vi "TIFF File Reader (LAVA.org).vi"(0 "Input Image":string) -> (3 "Grayscale":picture, 4 "Gray16/32":sgl[][](array[numeric]), 5 "Gray8":u8[][](array[numeric]), 7 "Gray u16":u16[][](array[numeric]))   [LabVIEW 2014]
doc: "This SubVI is an optimized version of the VI Load Flattened Image from Tiff.vi created by Gavin Burnell and Herbert Looser\n\nFiles in this folder downloaded from http://code.google.com/p/lavacr/source/browse/#svn/trunk/8.5.x/Machine%20Vision%20and%20Imaging/TIFF%20File%20Reader (free download).\nSee the discussion on https://lavag.org/topic/7170-tiff-reader/, where the link to above repository was provided.\nPeter Buerki, January 19, 2015."
uses:
  SubVIs/Globals.vi
  LAVA TIFF File Reader.lvlib
panel:
  out "Post View Image (NO IMAQ)":sgl[][](graph)
  in  "Tab Control":T1(tab)
  out "N_Bits":u64
  out "GrayWithLUT":picture
  out "Gray8 LUT":u8[][](array[numeric])
  out "RGB":picture
  out "N_RGB_Bits":u64
  out "R16/32":sgl[][](array[numeric])
  out "G16/32":sgl[][](array[numeric])
  out "B16/32":sgl[][](array[numeric])
  out "RGB8":u32[][](array[numeric])
  out "PhotoM":T2(ring)=enum."BlackIsZero"
  # "HD1:\\Users\\herbertlooser\\Desktop\\LadungssprŸher.tif"
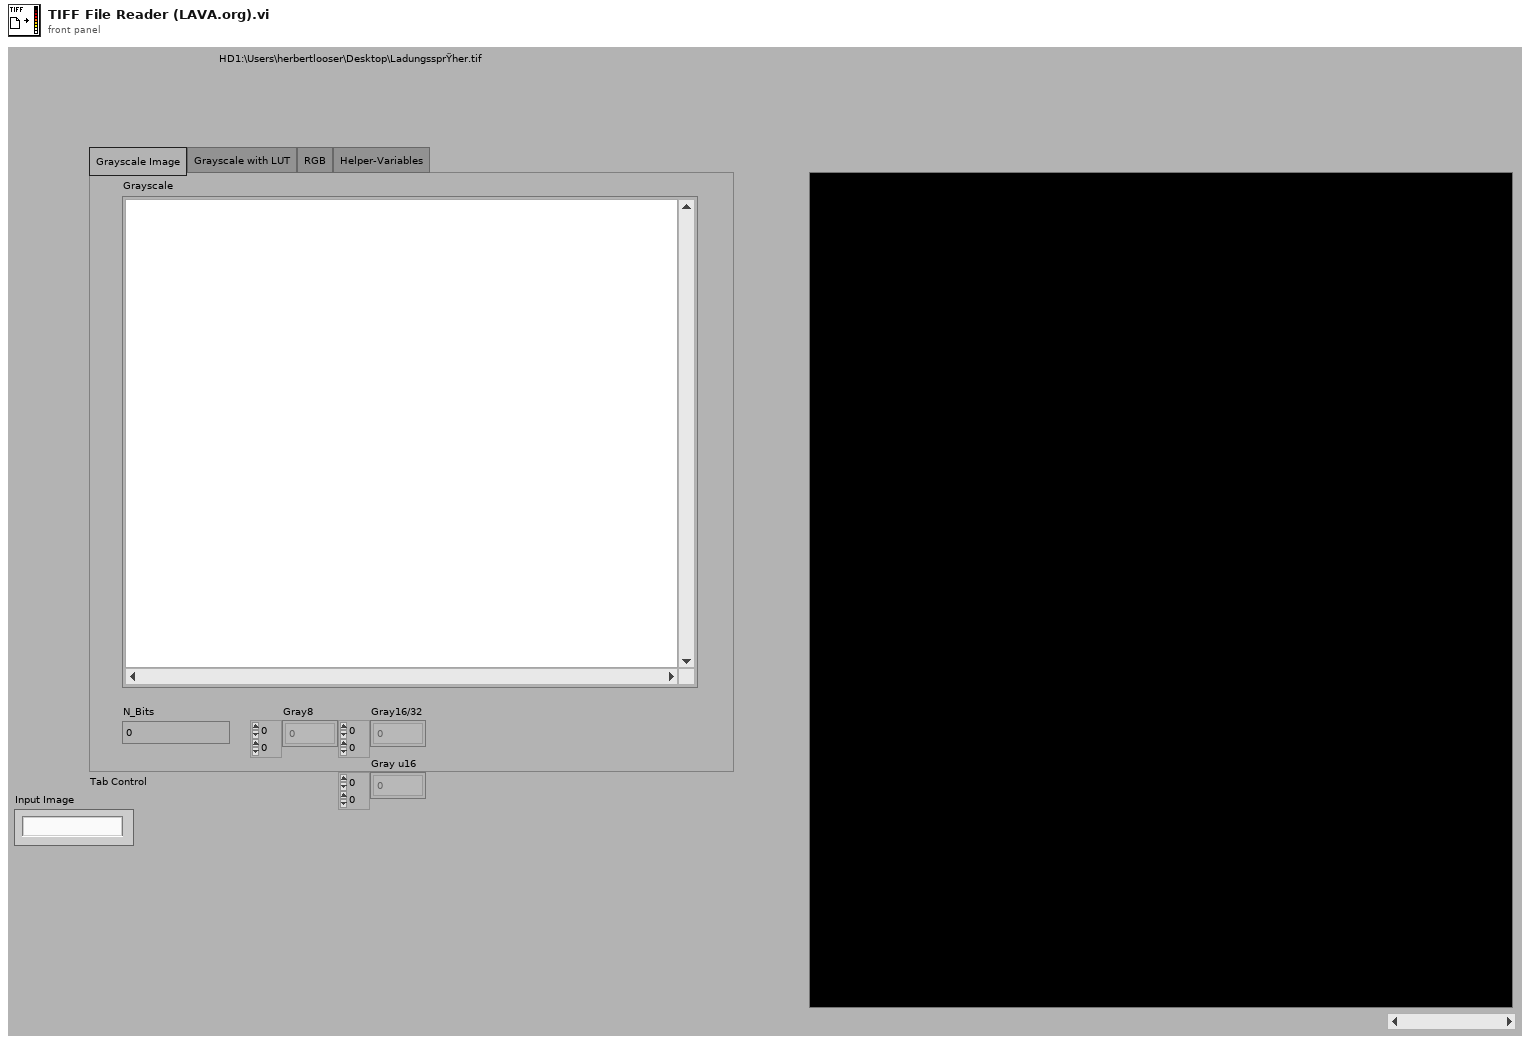
[diagram p1: front panel]
types:
  T1 = enum32{"Grayscale Image", "Grayscale with LUT", "RGB", "Helper-Variables"}
  T2 = enum16{"WhiteIsZero", "BlackIsZero", "RGB", "RGBPalette", "TranspMask", "CMYK", "YCbCr", "Null", "CIELab"}
  T3 = typedef "LAVA TIFF File Reader.lvlib/IFD Entry.ctl" = cluster{"Tag":u16, "Type":T4, "Count":u32, "Val/Offs":u32, "Is Val/Offs(T)":bool}
  T4 = typedef "LAVA TIFF File Reader.lvlib/FieldTypes.ctl" = enum16{"NULL", "U8", "ASCII7", "U16", "U32", "RATIONAL", "SByte(I8)", "Undef(8Bit)", "I16", "I32", "SRat(4B:4B)", "SGL(4Byte)", "DBL(8Byte)"}
  T5 = typedef "imagedata.ctl" = cluster{"image type":i32, "image depth":i32, "image":u8[], "mask":u8[], "colors":u32[], "Rectangle":cluster{"left":i16, "top":i16, "right":i16, "bottom":i16}}
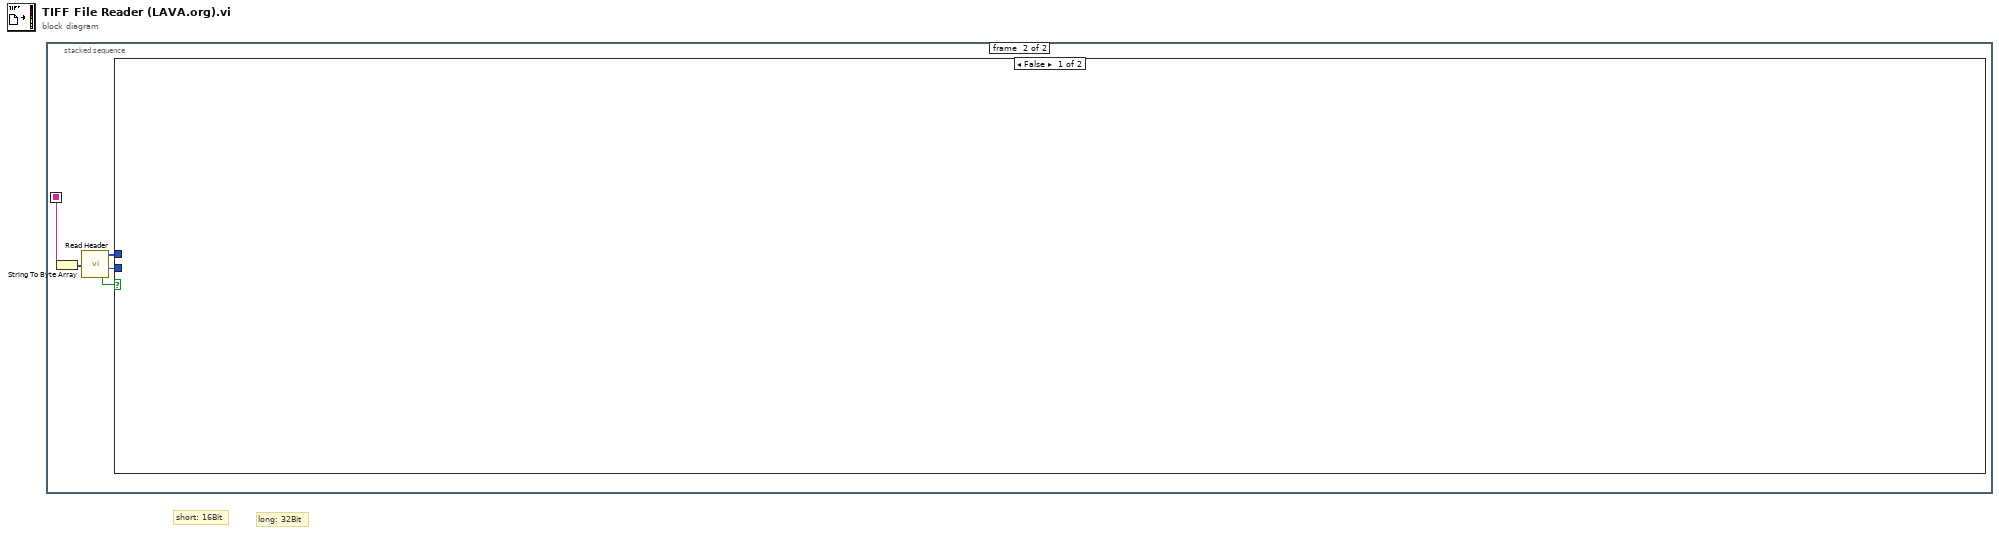
[diagram p0: block diagram]
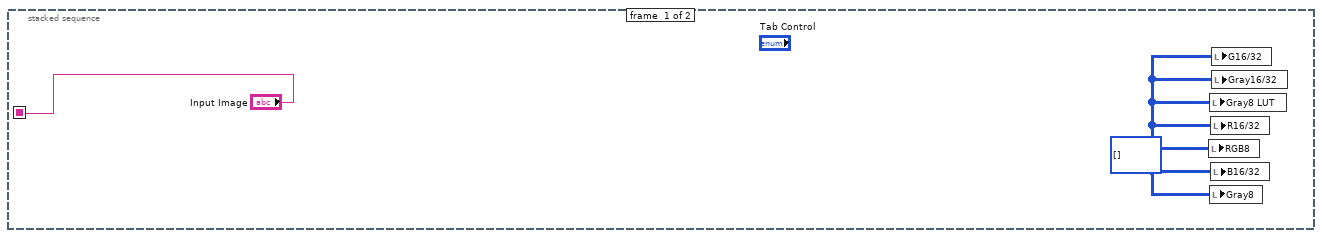
[diagram p2: hidden frame]
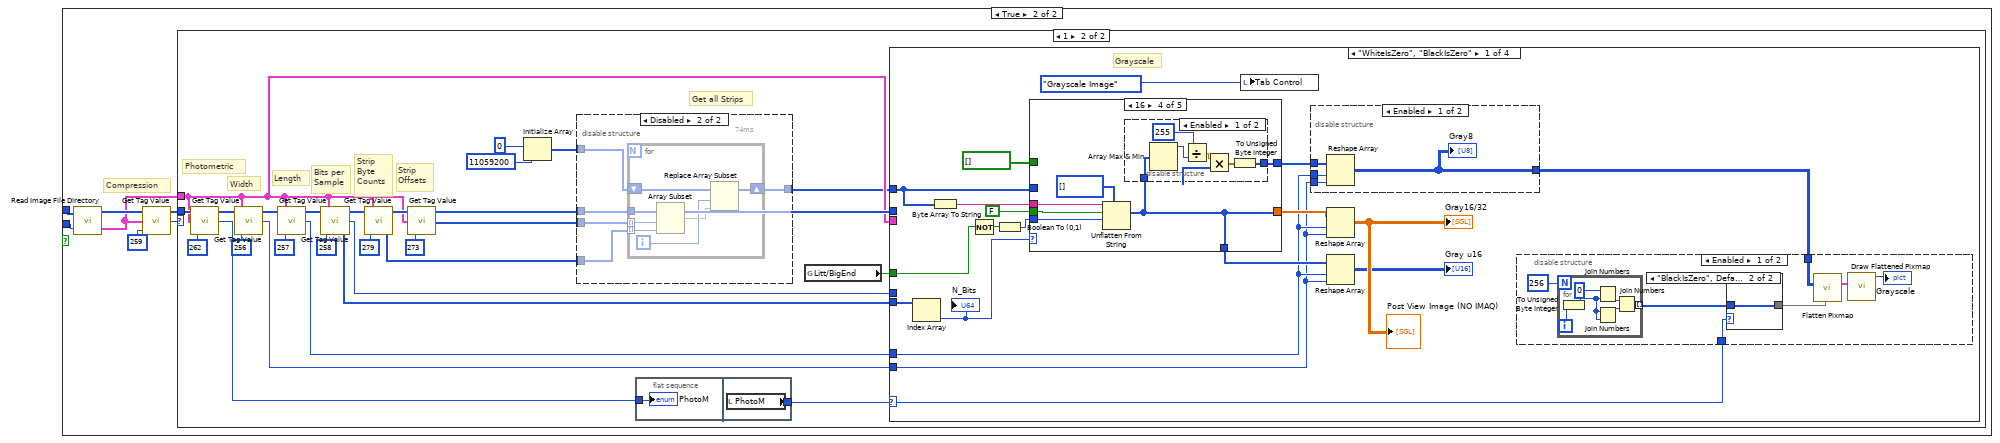
[diagram p3: hidden frame]
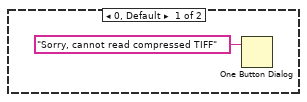
[diagram p4: hidden frame]
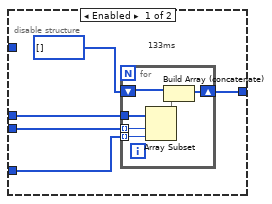
[diagram p5: hidden frame]
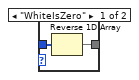
[diagram p7: hidden frame]
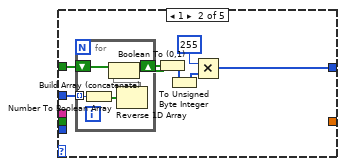
[diagram p10: hidden frame]
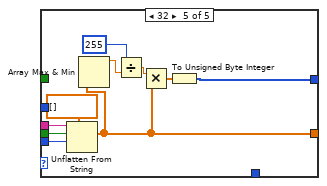
[diagram p13: hidden frame]
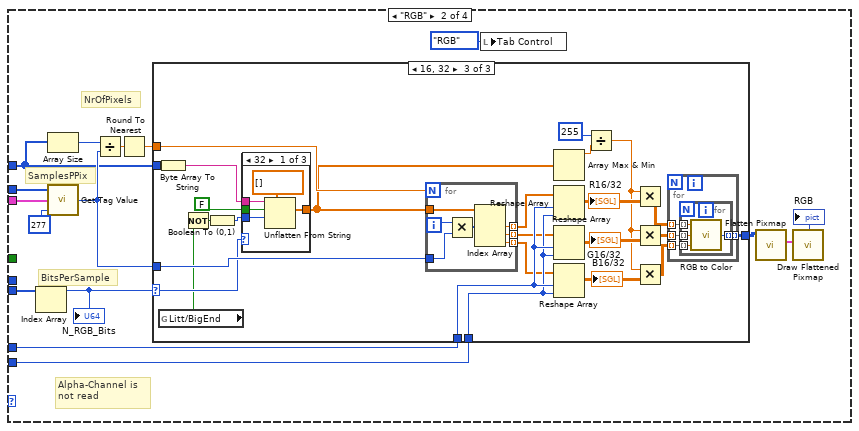
[diagram p14: hidden frame]
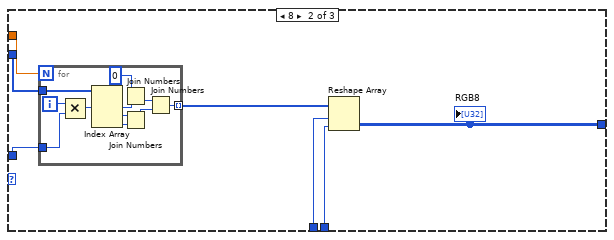
[diagram p16: hidden frame]
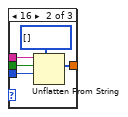
[diagram p17: hidden frame]
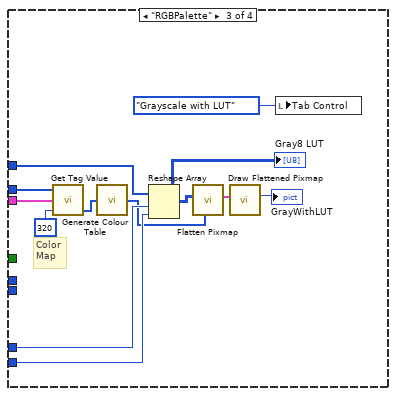
[diagram p19: hidden frame]
diagram:
  # "long: 32Bit"
  # "short: 16Bit"
  n1 = stacked-sequence {
    seq-local: ["Input Image" _] -> [_ w6]
    frame #0 {
      w2 = u32[][] [] ("RGB8")
      n2 = local write "RGB8"(w2) -> ()
      n3 = local write "Gray8 LUT"(w2) -> ()
      n4 = local write "Gray8"(w2) -> ()
      n5 = local write "R16/32"(w2) -> ()
      n6 = local write "B16/32"(w2) -> ()
      n7 = local write "G16/32"(w2) -> ()
      n8 = local write "Gray16/32"(w2) -> ()
    }
    frame #1 {
      n9 = String To Byte Array(string=w6) -> (unsigned byte array=w7:u8[])
      n10 = call "Read Header.vi"("Image Data in"=w7) -> ("Image Data out"=w5:u8[], "ImFileDirectOffs"=w4:u32, "isTIFF"=w3:bool)  [unwired: 1 in]
      n11 = case shown="False" w3 {
        tunnel: w5 -> [_ w13]
        tunnel: w4 -> [_ w12]
        frame False {
        }
        frame True {
          # "Compression"
          n12 = call "Read Image File Directory.vi"("Im_File_Dir Offs"=w12, "Image Data in"=w13) -> ("Directory"=w8:T3[], "Image Data out"=w11:u8[])
          n13 = call "Get Tag Value.vi"("Tag Code"=u16 259, "DirEntries"=w8) -> ("Single Value"=w9:u32)  [unwired: 1 in, 2 out]
          n14 = case shown="1" w9 {
            tunnel: w11 -> [_ w36]
            tunnel: w8 -> [_ w20]
            frame 0, Default {
              n15 = One Button Dialog(message="Sorry, cannot read compressed TIFF") -> ()  [unwired: 1 in, 1 out]
            }
            frame 1 {
              # "Get all Strips"
              # "Strip\nOffsets"
              # "Strip\nByte\nCounts"
              # "Bits per\nSample"
              # "Photometric"
              # "Length"
              # "Width"
              n16 = call "Get Tag Value.vi"("Tag Code"=u16 262, "DirEntries"=w20, "Image Data in"=w36) -> ("Single Value"=w25:u32, "Image Data out"=w35:u8[])  [unwired: 1 out]
              n17 = call "Get Tag Value.vi"("Tag Code"=u16 256, "DirEntries"=w20, "Image Data in"=w35) -> ("Single Value"=w37:u32, "Image Data out"=w41:u8[])  [unwired: 1 out]
              n18 = call "Get Tag Value.vi"("Tag Code"=u16 257, "DirEntries"=w20, "Image Data in"=w41) -> ("Single Value"=w38:u32, "Image Data out"=w32:u8[])  [unwired: 1 out]
              n19 = call "Get Tag Value.vi"("Tag Code"=u16 258, "DirEntries"=w20, "Image Data in"=w32) -> ("Multiple Values"=w26:u64[], "Single Value"=w27:u32, "Image Data out"=w31:u8[])
              n20 = call "Get Tag Value.vi"("Tag Code"=u16 279, "DirEntries"=w20, "Image Data in"=w31) -> ("Multiple Values"=w21:u64[], "Image Data out"=w30:u8[])  [unwired: 1 out]
              n21 = call "Get Tag Value.vi"("Tag Code"=u16 273, "DirEntries"=w20, "Image Data in"=w30) -> ("Multiple Values"=w22:u64[], "Image Data out"=w23:u8[])  [unwired: 1 out]
              n22 = Initialize Array(u8 0 ("Numeric"), 11059200 ("dimension size")) -> (w16:u8[])
              n23 = disable-structure shown="Disabled" {
                disable-tunnel: w23 -> [w46 w57]
                disable-tunnel: w22 -> [w45 w56]
                disable-tunnel: w21 -> [w44 w55]
                disable-tunnel: [w42 w54] -> w18
                disable-tunnel: w16 -> [_ w53]
                frame Enabled {
                  # "133ms"
                  n24 = for {
                    tunnel: w46 -> [w52]
                    tunnel: w45 -> [w51] mode=indexing
                    tunnel: w44 -> [w50] mode=indexing
                    shift-right: [w49] -> w42
                    shift-left: u8[] [] -> [w47]
                    n25 = Array Subset(array=w52, index=w51, length=w50) -> (w48:u8[])
                    n26 = Build Array (concatenate)(w47, w48) -> (w49:u8[])
                  }
                }
                frame Disabled {
                  # "74ms"
                  n27 = for {
                    tunnel: w57 -> [w64]
                    tunnel: w56 -> [w63] mode=indexing
                    tunnel: w55 -> [w62] mode=indexing
                    shift-right: [w60] -> w54
                    shift-left: w53 -> [w61]
                    i -> [w59]
                    n28 = Array Subset(array=w64, index=w63, length=w62) -> (w58:u8[])
                    n29 = Replace Array Subset(array=w61, new element=w58, index=w59) -> (w60:u8[])
                  }
                }
              }
              n30 = flat-sequence {
                tunnel: w25 -> [w65]
                tunnel: [w66] -> w24
                frame #0 {
                  "PhotoM" <- w65
                }
                frame #1 {
                  n31 = local read "PhotoM"() -> (w66:T2)
                }
              }
              n32 = global read "Globals.vi" "Litt/BigEnd"() -> (w19:bool)
              n33 = case shown="\"WhiteIsZero\", \"BlackIsZero\"" w24 {
                selector: w24 -> [w77 _ _ _]
                tunnel: w38 -> [w68 w156 w231 _]
                tunnel: w23 -> [_ w154 w233 _]
                tunnel: w37 -> [w67 w155 w230 _]
                tunnel: w20 -> [_ w153 w236 _]
                tunnel: w27 -> [_ _ _ _]
                tunnel: w26 -> [w81 w151 _ _]
                tunnel: w18 -> [w80 w142 w229 _]
                tunnel: w19 -> [w74 _ _ _]
                frame "WhiteIsZero", "BlackIsZero" {
                  # "Grayscale"
                  n34 = Index Array(array=w81) -> (element=w76:u64)  [unwired: 1 in]
                  "N_Bits" <- w76
                  n35 = Byte Array To String(unsigned byte array=w80) -> (string=w85:string)
                  n36 = Not(x=w74) -> (.not. x?=w82:bool)
                  n37 = Boolean To (0,1)(Boolean=w82) -> (0, 1=w83:i16)
                  n38 = case shown="16" w76 {
                    tunnel: w85 -> [_ _ _ w124 w139]
                    tunnel: [_ _ w118 w119 w132] -> w78
                    tunnel: FALSE ("data includes array or string size? (T)") -> [_ _ _ w123 w138]
                    tunnel: w83 -> [_ _ _ w122 w137]
                    tunnel: w80 -> [_ w112 w118 _ _]
                    tunnel: [_ w107 w118 w120 w133] -> w79
                    tunnel: bool[] [] -> [_ w106 _ _ _]
                    tunnel: [_ _ _ w119 _] -> w69
                    frame 0, 4, Default {
                      # "not\nsupported"
                    }
                    frame 1 {
                      n39 = for {
                        tunnel: w112 -> [w117] mode=indexing
                        shift-right: [w116] -> w111
                        shift-left: w106 -> [w115]
                        n40 = Number To Boolean Array(number=w117) -> (Boolean array=w114:bool[])
                        n41 = Reverse 1D Array(array=w114) -> (reversed array=w113:bool[])
                        n42 = Build Array (concatenate)(w115, w113) -> (w116:bool[])
                      }
                      n43 = Boolean To (0,1)(Boolean=w111) -> (0, 1=w110:i16[])
                      n44 = To Unsigned Byte Integer(number=w110) -> (unsigned 8bit integer=w109:u8[])
                      n45 = Multiply(x=u8 255, y=w109) -> (x*y=w107:u8[])
                    }
                    frame 8 {
                    }
                    frame 16 {
                      n46 = Unflatten From String(type=u16[] [], binary string=w124, data includes array or string size? (T)=w123, byte order (0:big-endian, network order)=w122) -> (value=w119:u16[])  [unwired: 1 in, 2 out]
                      n47 = disable-structure shown="Enabled" {
                        disable-tunnel: [w126 _] -> w120
                        disable-tunnel: w119 -> [w125 _]
                        frame Enabled {
                          n48 = Array Max & Min(array=w125) -> (max value=w130:u16)  [unwired: 3 out]
                          n49 = Divide(x=255 ("Numeric"), y=w130) -> (x/y=w129:dbl)
                          n50 = Multiply(x=w129, y=w125) -> (x*y=w127:dbl[])
                          n51 = To Unsigned Byte Integer(number=w127) -> (unsigned 8bit integer=w126:u8[])
                        }
                        frame Disabled {
                        }
                      }
                    }
                    frame 32 {
                      n52 = Unflatten From String(type=sgl[] [], binary string=w139, data includes array or string size? (T)=w138, byte order (0:big-endian, network order)=w137) -> (value=w132:sgl[])  [unwired: 1 in, 2 out]
                      n53 = Array Max & Min(array=w132) -> (max value=w136:sgl)  [unwired: 3 out]
                      n54 = Divide(x=255 ("Numeric"), y=w136) -> (x/y=w135:sgl)
                      n55 = Multiply(x=w135, y=w132) -> (x*y=w134:sgl[])
                      n56 = To Unsigned Byte Integer(number=w134) -> (unsigned 8bit integer=w133:u8[])
                    }
                  }
                  n57 = local write "Tab Control"(T1."Grayscale Image" ("Tab Control")) -> ()
                  n58 = disable-structure shown="Enabled" {
                    disable-tunnel: w79 -> [w89 _]
                    disable-tunnel: w68 -> [w88 _]
                    disable-tunnel: w67 -> [w87 _]
                    disable-tunnel: [w86 _] -> w72
                    frame Enabled {
                      n59 = Reshape Array(w89, w88, w87) -> (w86:u8[][])
                      "Gray8" <- w86
                    }
                    frame Disabled {
                    }
                  }
                  n60 = Reshape Array(w78, w68, w67) -> (→"Gray16/32" →"Post View Image (NO IMAQ)":sgl[][])
                  n61 = Reshape Array(w69, w68, w67) -> (→"Gray u16":u16[][])
                  n62 = disable-structure shown="Enabled" {
                    disable-tunnel: w77 -> [w92 _]
                    disable-tunnel: w72 -> [w90 _]
                    frame Enabled {
                      n63 = for {
                        N: 256 -> [_]
                        tunnel: [w100] -> w94 mode=indexing
                        i -> [w105]
                        n64 = To Unsigned Byte Integer(number=w105) -> (unsigned 8bit integer=w103:u8)
                        n65 = Join Numbers(hi=u8 0, lo=w103) -> ((hi.lo)=w101:u16)
                        n66 = Join Numbers(hi=w103, lo=w103) -> ((hi.lo)=w102:u16)
                        n67 = Join Numbers(hi=w101, lo=w102) -> ((hi.lo)=w100:u32)
                      }
                      n68 = case shown="\"BlackIsZero\", Default" w92 {
                        tunnel: w94 -> [w98 w99]
                        tunnel: [w97 w99] -> w93
                        frame "WhiteIsZero" {
                          n69 = Reverse 1D Array(array=w98) -> (reversed array=w97:u32[])
                        }
                        frame "BlackIsZero", Default {
                        }
                      }
                      n70 = call <vilib>:"Flatten Pixmap.vi"("colors"=w93, "8-bit pixmap"=w90) -> ("image data"=w96:T5)  [unwired: 9 in]
                      n71 = call <vilib>:"Draw Flattened Pixmap.vi"("image data"=w96) -> ("new picture"=→"Grayscale":picture)  [unwired: 8 in]
                    }
                    frame Disabled {
                    }
                  }
                }
                frame "RGB" {
                  # "BitsPerSample"
                  # "NrOfPixels"
                  # "Alpha-Channel is\nnot read"
                  # "SamplesPPix"
                  n72 = Index Array(array=w151) -> (element=w146:u64)  [unwired: 1 in]
                  "N_RGB_Bits" <- w146
                  n73 = Array Size(array=w142) -> (size(s)=w141:i32)
                  n74 = call "Get Tag Value.vi"("Tag Code"=u16 277, "DirEntries"=w153, "Image Data in"=w154) -> ("Single Value"=w148:u32)  [unwired: 2 out]
                  n75 = Divide(x=w141, y=w148) -> (x/y=w150:dbl)
                  n76 = Round To Nearest(number=w150) -> (nearest integer value=w149:dbl)
                  n77 = case shown="16, 32" w146 {
                    selector: w146 -> [_ _ w191]
                    tunnel: w156 -> [_ w162 w199]
                    tunnel: w155 -> [_ w161 w198]
                    tunnel: w148 -> [_ w160 w195]
                    tunnel: w142 -> [_ w159 w190]
                    tunnel: w149 -> [_ w158 w196]
                    tunnel: [_ w157 w176] -> w143
                    frame 0, Default {
                    }
                    frame 8 {
                      n78 = for {
                        N: w158 -> [_]
                        tunnel: w159 -> [w174]
                        tunnel: [w167] -> w163 mode=indexing
                        tunnel: w160 -> [w164]
                        i -> [w165]
                        n79 = Multiply(x=w165, y=w164) -> (x*y=w166:u32)
                        n80 = Index Array(array=w174, index #1=w166) -> (element #1=w173:u8, element #2=w172:u8, element #3=w171:u8)  [unwired: 2 in]
                        n81 = Join Numbers(hi=u8 0, lo=w173) -> ((hi.lo)=w168:u16)
                        n82 = Join Numbers(hi=w172, lo=w171) -> ((hi.lo)=w169:u16)
                        n83 = Join Numbers(hi=w168, lo=w169) -> ((hi.lo)=w167:u32)
                      }
                      n84 = Reshape Array(w163, w162, w161) -> (w157:u32[][])
                      "RGB8" <- w157
                    }
                    frame 16, 32 {
                      n85 = Byte Array To String(unsigned byte array=w190) -> (string=w197:string)
                      n86 = global read "Globals.vi" "Litt/BigEnd"() -> (w175:bool)
                      n87 = Not(x=w175) -> (.not. x?=w192:bool)
                      n88 = Boolean To (0,1)(Boolean=w192) -> (0, 1=w193:i16)
                      n89 = case shown="32" w191 {
                        tunnel: w197 -> [w212 w217 _]
                        tunnel: [w208 w216 _] -> w186
                        tunnel: FALSE ("data includes array or string size? (T)") -> [w211 w215 _]
                        tunnel: w193 -> [w210 w214 _]
                        frame 32 {
                          n90 = Unflatten From String(type=sgl[] [], binary string=w212, data includes array or string size? (T)=w211, byte order (0:big-endian, network order)=w210) -> (value=w208:sgl[])  [unwired: 1 in, 2 out]
                        }
                        frame 16 {
                          n91 = Unflatten From String(type=u16[] [], binary string=w217, data includes array or string size? (T)=w215, byte order (0:big-endian, network order)=w214) -> (value=w216:u16[])  [unwired: 1 in, 2 out]
                        }
                        frame 0, Default {
                        }
                      }
                      n92 = for {
                        N: w196 -> [_]
                        tunnel: w186 -> [w224]
                        tunnel: [w223] -> w185 mode=indexing
                        tunnel: [w222] -> w189 mode=indexing
                        tunnel: [w221] -> w188 mode=indexing
                        tunnel: w195 -> [w218]
                        i -> [w219]
                        n93 = Multiply(x=w219, y=w218) -> (x*y=w220:u32)
                        n94 = Index Array(array=w224, index #1=w220) -> (element #1=w223:sgl, element #2=w222:sgl, element #3=w221:sgl)  [unwired: 2 in]
                      }
                      n95 = Array Max & Min(array=w186) -> (max value=w184:sgl)  [unwired: 3 out]
                      n96 = Reshape Array(w185, w199, w198) -> (w183:sgl[][])
                      "R16/32" <- w183
                      n97 = Reshape Array(w189, w199, w198) -> (w182:sgl[][])
                      "G16/32" <- w182
                      n98 = Reshape Array(w188, w199, w198) -> (w181:sgl[][])
                      "B16/32" <- w181
                      n99 = Divide(x=255, y=w184) -> (x/y=w180:sgl)
                      n100 = Multiply(x=w180, y=w183) -> (x*y=w179:sgl[][])
                      n101 = Multiply(x=w180, y=w182) -> (x*y=w178:sgl[][])
                      n102 = Multiply(x=w180, y=w181) -> (x*y=w177:sgl[][])
                      n103 = for {
                        tunnel: w179 -> [w203] mode=indexing
                        tunnel: w178 -> [w202] mode=indexing
                        tunnel: w177 -> [w201] mode=indexing
                        tunnel: [w200] -> w176 mode=indexing
                        n104 = for {
                          tunnel: w203 -> [w207] mode=indexing
                          tunnel: w202 -> [w206] mode=indexing
                          tunnel: w201 -> [w205] mode=indexing
                          tunnel: [w204] -> w200 mode=indexing
                          n105 = call <vilib>:"RGB to Color.vi"("B"=w205, "G"=w206, "R"=w207) -> ("Color"=w204:u32)
                        }
                      }
                    }
                  }
                  n106 = local write "Tab Control"(T1."RGB" ("Tab Control")) -> ()
                  n107 = call <vilib>:"Flatten Pixmap.vi"("24-bit pixmap"=w143) -> ("image data"=w144:T5)  [unwired: 10 in]
                  n108 = call <vilib>:"Draw Flattened Pixmap.vi"("image data"=w144) -> ("new picture"=→"RGB":picture)  [unwired: 8 in]
                }
                frame "RGBPalette" {
                  # "Color\nMap"
                  n109 = call "Get Tag Value.vi"("Tag Code"=u16 320, "DirEntries"=w236, "Image Data in"=w233) -> ("Multiple Values"=w235:u64[])  [unwired: 2 out]
                  n110 = call "Generate Colour Table.vi"("Code 320 Values"=w235) -> ("Colour Table"=w228:u32[])
                  n111 = Reshape Array(w229, w231, w230) -> (w225:u8[][])
                  "Gray8 LUT" <- w225
                  n112 = call <vilib>:"Flatten Pixmap.vi"("colors"=w228, "8-bit pixmap"=w225) -> ("image data"=w232:T5)  [unwired: 9 in]
                  n113 = call <vilib>:"Draw Flattened Pixmap.vi"("image data"=w232) -> ("new picture"=→"GrayWithLUT":picture)  [unwired: 8 in]
                  n114 = local write "Tab Control"(T1."Grayscale with LUT" ("Tab Control")) -> ()
                }
                frame "TranspMask".."CIELab" {
                  # "unsupported"
                }
              }
            }
          }
        }
      }
    }
  }
